vi "相机1-分析PCB孔影像-校准和自动共用.vi"(8 "error in (no error)":errorcluster, 9 "拍照功能":T10, 10 "取像时间":u32, 11 "Image In":T12) -> (0 "error out":errorcluster, 1 "Mark点拍照结果":bool=TRUE, 2 "mark Angle":sgl, 3 "Image":T12(plugin-control), 4 "存档数据和结果 out":T9={"待写入数据"=[], "单个结果"=[], "总结果"=FALSE, "数据有效"=TRUE}, 5 "视觉补偿机械手移动量 mm":T11 {"X" format="%#.3f"})   [LabVIEW 2014]
uses:
  <vilib>/vision/Image Controls.llb/IMAQ Image.ctl
  Controls/XYPos.ctl
  <vilib>/vision/Instrument.llb/QR Code Report.ctl
  <vilib>/vision/Instrument.llb/QR Code Model Type.ctl
  <vilib>/vision/Instrument.llb/QR Code Stream Mode Type.ctl
  <vilib>/vision/Instrument.llb/Data Matrix Polarity.ctl
  <vilib>/vision/Instrument.llb/Demodulation Mode.ctl
  <vilib>/vision/Instrument.llb/Cell Sample Size.ctl
  <vilib>/vision/Instrument.llb/Cell Filter Mode.ctl
  Controls/TestThreshold.ctl
  <vilib>/vision/Measure.llb/Edge Options.ctl
  <vilib>/vision/Measure.llb/Edge Polarity.ctl
  Global.vi
  <vilib>/vision/NI_Vision_Development_Module.lvlib
panel:
  out "QR Barcode Report (2D Barcode Reader 1)":T1={"Found?"=FALSE, "Data"="", "Bounding Box"=[], "Errors Corrected"=0, "Dimensions (Rows/Cols)"=0, "Version"=0, "QR Model"=3, "Stream Mode"=0, "Barcode Polarity"=-2, "Mirrored?"=FALSE, "Append Stream Position"=0, "Size of Append Stream"=0, "First EAN-128 ID"=0, "First Alternate Language ID"=0, "Append Stream ID"=0, "Minimum Edge Strength"=30, "Demodulation Mode"=-2, "Cell Sample Size"=-2, "Cell Filter Mode"=-2} {"Append Stream ID" format="%x"; "Cell Filter Mode" items=["Auto-detect"=-2, "Average"=0, "Median"=1, "Central Average"=2, "High Average"=3, "Low Average"=4, "Very High Average"=5, "Very Low Average"=6, "All Filters"=8]; "Cell Sample Size" items=["Auto-detect"=-2, "1x1"=1, "2x2"=2, "3x3"=3, "4x4"=4, "5x5"=5, "6x6"=6, "7x7"=7]; "Demodulation Mode" items=["Auto-detect"=-2, "Histogram"=0, "Local Contrast"=1, "Combination"=2, "All"=3]; "Barcode Polarity" items=["Auto-detect"=-2, "Black on White"=0, "White on Black"=1]; "Stream Mode" items=["Auto-detect", "Numeric", "AlphaNumeric", "Mixed", "Raw Bytes", "UCC/EAN-128 - In Tokens", "UCC/EAN-128 - In Data", "Extended Character Interpretation", "Kanji"]; "QR Model" items=["Auto Detect", "Micro", "Model 1", "Model 2"]; "Version" max=40 step=1}
  out "Fitted Circle 2":T8 {"Average SNR (dB)" format="%.2f"; "Average Strength" format="%.2f"; "Roundness (Real-World)" format="%.2f"; "Radius (Real-World)" format="%.2f"; "Center (Real-World)"."Y" format="%.2f"; "Center (Real-World)"."X" format="%.2f"; "Radius (Pixels)" format="%.2f"; "Center (Pixels)"."Y" format="%.2f"; "Center (Pixels)"."X" format="%.2f"}
  out "Fitted Circle":T8 {"Average SNR (dB)" format="%.2f"; "Average Strength" format="%.2f"; "Roundness (Real-World)" format="%.2f"; "Radius (Real-World)" format="%.2f"; "Center (Real-World)"."Y" format="%.2f"; "Center (Real-World)"."X" format="%.2f"; "Radius (Pixels)" format="%.2f"; "Center (Pixels)"."Y" format="%.2f"; "Center (Pixels)"."X" format="%.2f"}
  in  "存档数据和结果":T9={"待写入数据"=[], "单个结果"=[], "总结果"=FALSE, "数据有效"=TRUE}
  in  "显示内容 2":string[](array[string])=["补偿量-X", "补偿量-Y", "补偿量-角度"]
  out "图像偏差量Pixles":T11 {"X" format="%#.3f"}
  in  "Img Path":path=path "C:/Users/aicter/Desktop/上相机对位时Gold影像.png"
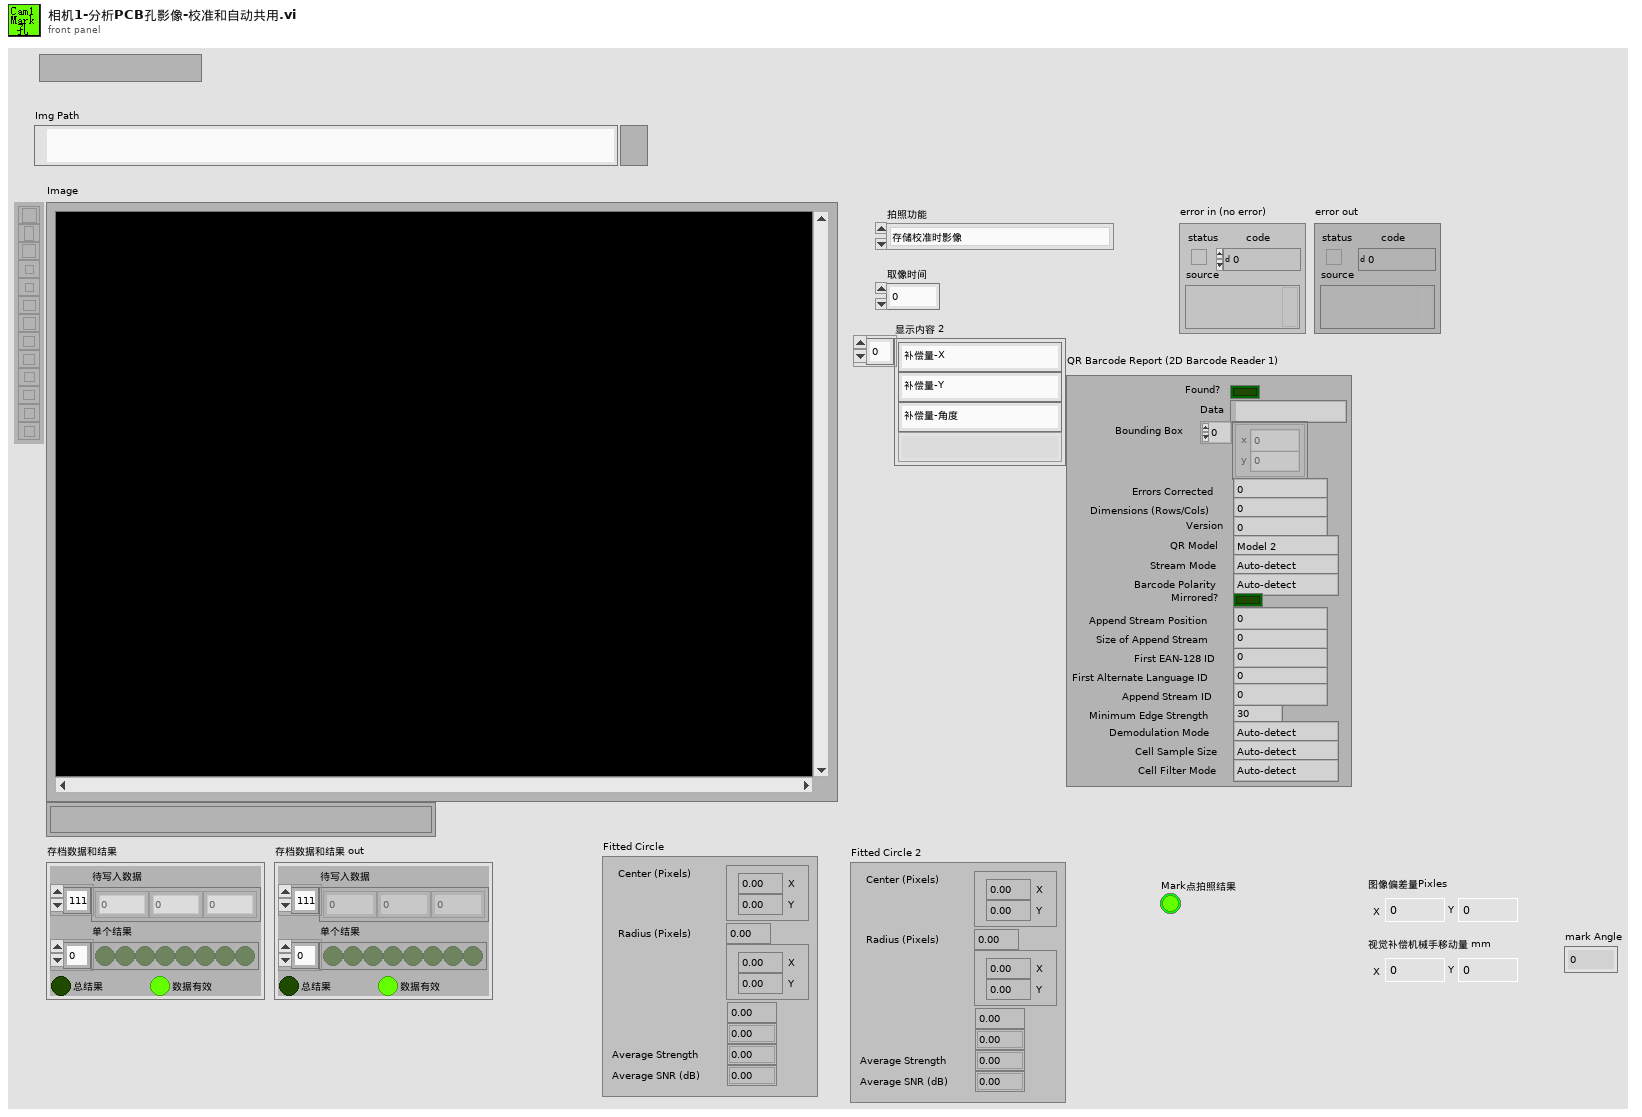
[diagram p1: front panel]
types:
  T1 = typedef "QR Code Report.ctl" = cluster{"Found?":bool, "Data":string, "Bounding Box":cluster{"x":sgl, "y":sgl}[], "Errors Corrected":u32, "Dimensions (Rows/Cols)":u32, "Version":u32, "QR Model":T2, "Stream Mode":T3, "Barcode Polarity":T4, "Mirrored?":bool, "Append Stream Position":u32, "Size of Append Stream":u32, "First EAN-128 ID":i32, "First Alternate Language ID":i32, "Append Stream ID":u32, "Minimum Edge Strength":u32, "Demodulation Mode":T5, "Cell Sample Size":T6, "Cell Filter Mode":T7}
  T2 = typedef "QR Code Model Type.ctl" = i32
  T3 = typedef "QR Code Stream Mode Type.ctl" = i32
  T4 = typedef "Data Matrix Polarity.ctl" = i32
  T5 = typedef "Demodulation Mode.ctl" = i32
  T6 = typedef "Cell Sample Size.ctl" = i32
  T7 = typedef "Cell Filter Mode.ctl" = i32
  T8 = cluster{"Center (Pixels)":cluster{"X":sgl, "Y":sgl}, "Radius (Pixels)":dbl, "Center (Real-World)":cluster{"X":sgl, "Y":sgl}, "Radius (Real-World)":dbl, "Roundness (Real-World)":dbl, "Average Strength":dbl, "Average SNR (dB)":dbl}
  T9 = typedef "存档数据和结果.ctl" = cluster{"待写入数据":dbl[], "单个结果":bool[], "总结果":bool, "数据有效":bool}
  T10 = typedef "控件-拍照PCB孔分类.ctl" = enum16{"存储校准时影像", "拍照孔-Mark1", "拍照孔-Mark2", "拍照二维码", "计算补偿量"}
  T11 = typedef "XYPos.ctl" = cluster{"X":dbl, "Y":dbl}
  T12 = typedef "IMAQ Image.ctl" = refnum<image>
  T13 = typedef "Edge Options.ctl" = cluster{"Edge Polarity":T14, "Kernel Size":u32, "Width":u32, "Minimum Edge Strength":sgl, "Interpolation Type":enum32{"Zero Order", "Bilinear", "Quadratic", "Cubic", "Bilinear Fixed"}, "Data Processing Method":enum32{"Average", "Median"}}
  T14 = typedef "Edge Polarity.ctl" = u32
  T15 = cluster{"Search  Direction":u32, "Edge Options":T13, "Show Search Area":bool, "Show Search Lines":bool, "Show Edges Found":bool, "Show Result":bool, "Search Area Color":u32, "Search Lines Color":u32, "Edge Locations Color":u32, "Result Color":u32, "Overlay Group Name":string}
  T16 = typedef "TestThreshold.ctl" = cluster{"下限":dbl, "上限":dbl}
  T17 = typedef "OtherSpec.ctl" = cluster{"其它勾选类规格":T18, "其它数据类规格":T19, "相机名称":T20, "参数":cluster{"Mark1曝光时间":i32, "Mark2曝光时间":i32, "二维码曝光时间":i32}}
  T18 = typedef "其它勾选类规格.ctl" = cluster{"保存图片":bool, "上传设备状态数据":bool, "保存数据":bool, "开机默认开启监控摄像头":bool, "启用mark拍照 ":bool}
  T19 = typedef "其他数据类规格.ctl" = cluster{"相机1像素-毫米换算系数":dbl, "相机2像素-毫米换算系数":dbl, "D盘剩余空间预警(G)":dbl, "视频最长录制时间(秒)":dbl}
  T20 = typedef "相机名称品牌使用状态.ctl" = cluster{"相机1名称":T21, "相机2名称":T21, "Cam1启用":bool, "Cam2启用":bool, "Basler1":bool, "Basler2":bool}
  T21 = typedef "IMAQdx.ctl" = refnum<k21>
  T22 = typedef "mark规格.ctl" = cluster{"X下限":dbl, "X上限":dbl, "Y下限":dbl, "Y 上限":dbl, "angle下限":dbl, "angle上限":dbl}
  T23 = cluster{"甩线补偿值":cluster{"下边":dbl, "距离上边":dbl, "左边":dbl, "右边":dbl}, "补偿甩线坐标偏移":T11, "mark点模组补偿":T11, "出线补偿值":dbl, "mark规格":T22}
  T24 = cluster{"mark 1 ":cluster{"X":dbl, "Y":dbl}, "mark 2":cluster{"X":dbl, "Y":dbl}}
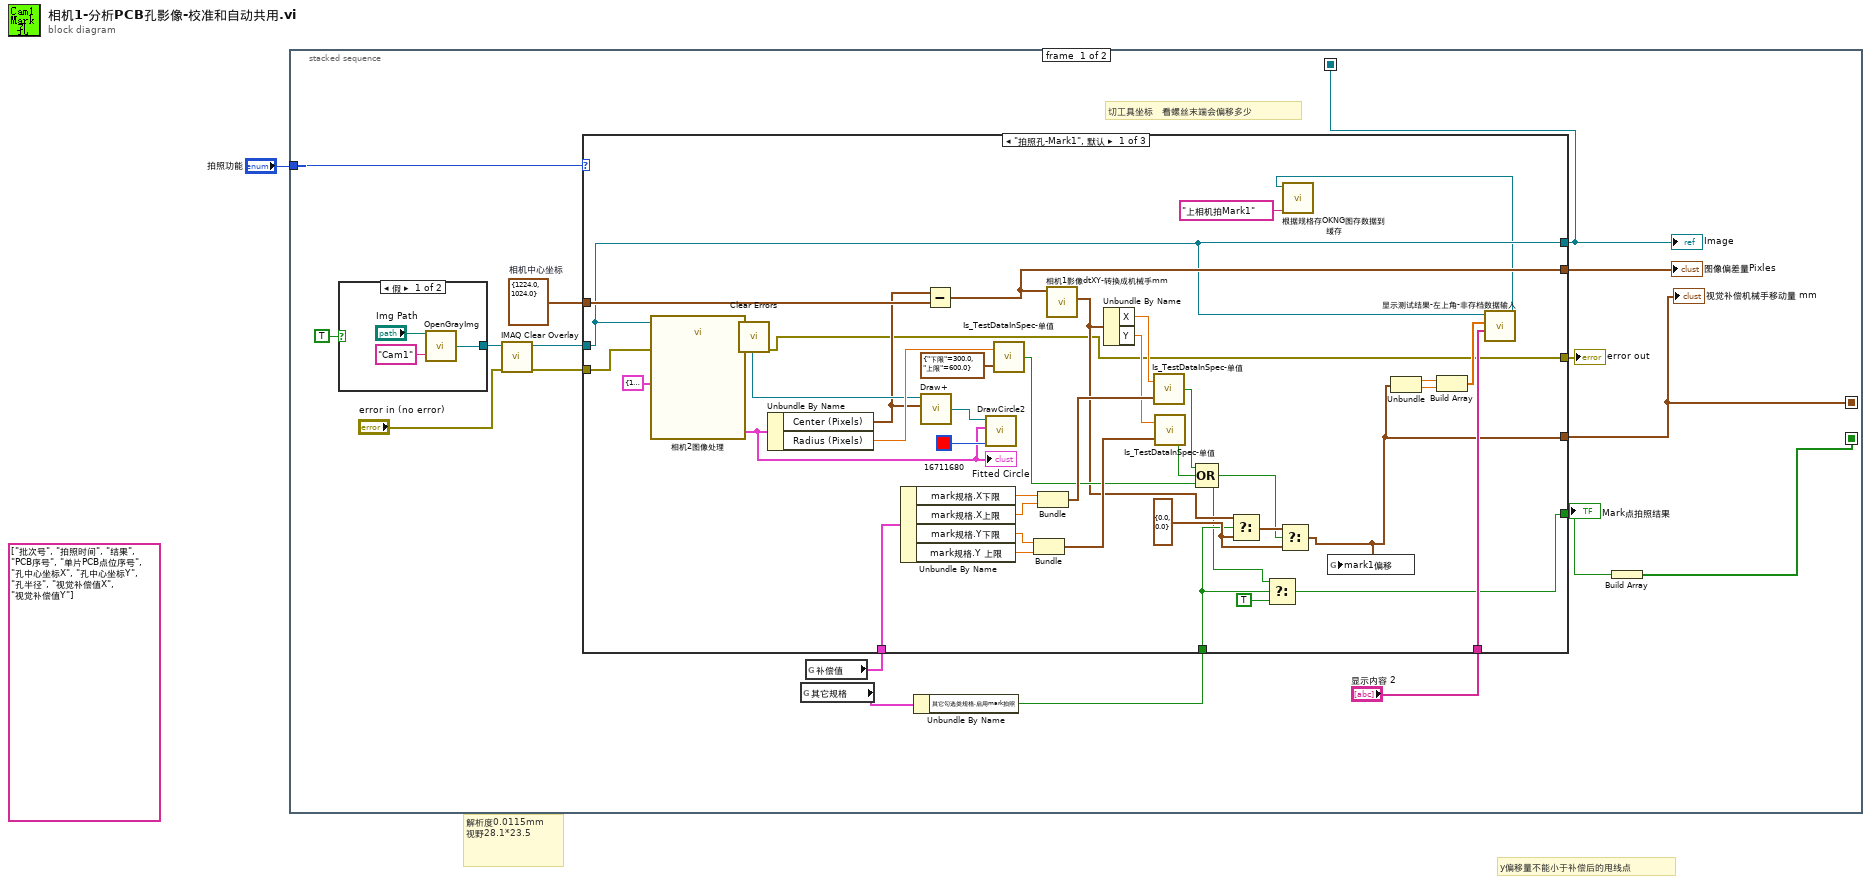
[diagram p0: block diagram]
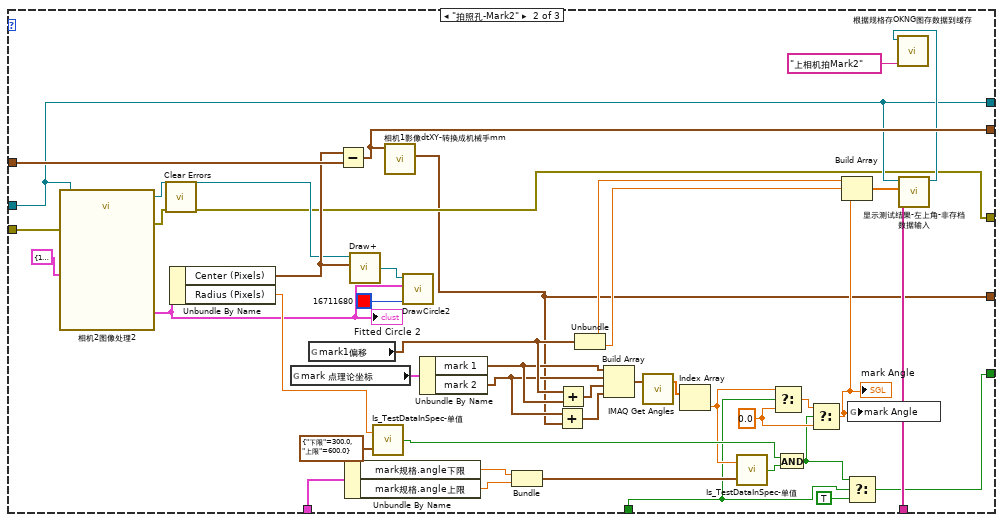
[diagram p2: hidden frame]
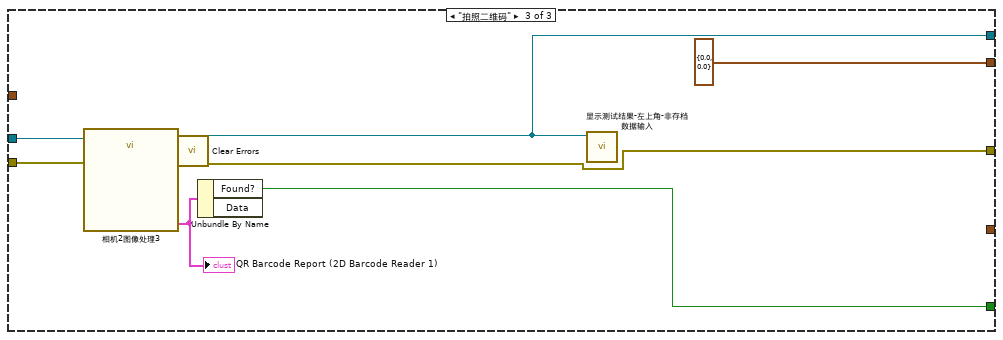
[diagram p3: hidden frame]
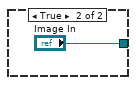
[diagram p4: hidden frame]
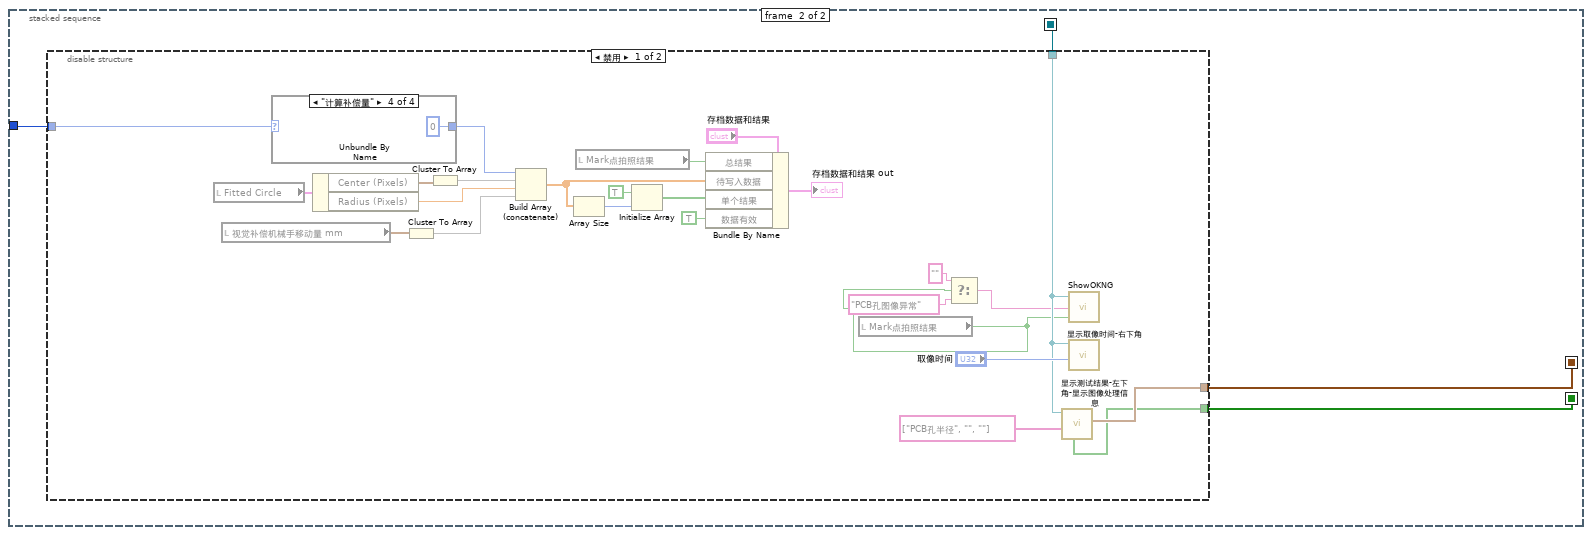
[diagram p5: hidden frame]
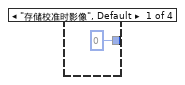
[diagram p6: hidden frame]
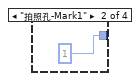
[diagram p7: hidden frame]
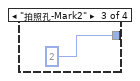
[diagram p8: hidden frame]
diagram:
  (unwired) string[] ["批次号", "拍照时间", "结果", "PCB序号", "单片PCB点位序号", "孔中心坐标X", "孔中心坐标Y", "孔半径", "视觉补偿值X", "视觉补偿值Y"] ("拍PCB孔信息")
  # "y偏移量不能小于补偿后的甩线点"
  # "解析度0.0115mm\n视野28.1*23.5"
  n1 = stacked-sequence {
    seq-local: [w13 _] -> [_ w116]
    seq-local: [w4 _] -> [_ w115]
    seq-local: [w12 _] -> [_ w114]
    tunnel: "拍照功能" -> [w14 w117]
    frame #0 {
      w16 = T11 {"X"=1224.0, "Y"=1024.0}  # 相机中心坐标
      # "切工具坐标   看螺丝末端会偏移多少"
      n2 = case shown="假" TRUE {
        tunnel: [w112 "Image In"] -> w18
        frame False {
          n3 = call "OpenGrayImg.vi"("Image Name"="Cam1", "Img Path"="Img Path") -> ("Image Out"=w112:T12)
        }
        frame True {
        }
      }
      n4 = call "IMAQ Clear Overlay"("error in (no error)"="error in (no error)", "Image"=w18) -> ("error out"=w8:errorcluster, "Image Out"=w7:T12)  [unwired: 8 in]
      n5 = global read "Global.vi" "其它规格"() -> (w11:T17)
      n6 = global read "Global.vi" "补偿值"() -> (w3:T23)
      n7 = Unbundle By Name(w11) -> ("其它勾选类规格.启用mark拍照"=w2:bool)
      n8 = case shown="\"拍照孔-Mark1\", 默认" w14 {
        tunnel: w7 -> [w48 w65 w108]
        tunnel: w16 -> [w58 w100 _]
        tunnel: [w48 w65 w105] -> w13
        tunnel: [w57 w99 T11 {"X"=0.0, "Y"=0.0} ("相机中心坐标")] -> w15
        tunnel: "显示内容 2" -> [w55 w97 _]
        tunnel: w8 -> [w46 w64 w109]
        tunnel: [w20 w60 w102] -> w6
        tunnel: [w23 w68 w103] -> w5
        tunnel: [w19 w59 _] -> w4
        tunnel: w3 -> [w32 w86 _]
        tunnel: w2 -> [w24 w70 _]
        frame "拍照孔-Mark1", Default {
          w29 = T11 {"X"=0.0, "Y"=0.0} ("f")
          n9 = call "相机2图像处理"("Image In"=w48, "Options (Find Circular Edge 1)"=T15 {"Search  Direction"=1, "Edge Options"={"Edge Polarity"=1, "Kernel Size"=9, "Width"=5, "Minimum Edge Strength"=30.0, "Interpolation Type"=enum."Bilinear Fixed", "Data Processing Method"=enum."Average"}, "Show Search Area"=FALSE, "Show Search Lines"=FALSE, "Show Edges Found"=TRUE, "Show Result"=FALSE, "Search Area Color"=65280, "Search Lines Color"=255, "Edge Locations Color"=16776960, "Result Color"=16711680, "Overlay Group Name"=""}, "error in"=w46) -> ("Image Out"=w47:T12, "Fitted Circle (Find Circular Edge 1)"=w52:T8, "error out"=w44:errorcluster)  [unwired: 21 in, 1 out]
          "Fitted Circle" <- w52
          n10 = call <vilib>:"Clear Errors.vi"("error in (no error)"=w44) -> ("error out"=w20:errorcluster)  [unwired: 5 in, 1 out]
          n11 = Unbundle By Name(w52) -> ("Center (Pixels)"=w45:cluster{"X":sgl, "Y":sgl}, "Radius (Pixels)"=w50:dbl)
          n12 = Unbundle By Name(w32) -> ("mark规格.X下限"=w42:dbl, "mark规格.X上限"=w41:dbl, "mark规格.Y下限"=w38:dbl, "mark规格.Y 上限"=w37:dbl)
          n13 = call "Draw+.vi"("input cluster"=w45, "Image In"=w47) -> ("Image Out"=w54:T12)  [unwired: 4 in]
          n14 = Subtract(x=w45, y=w58) -> (x-y=w57:T11)
          n15 = call "DrawCircle2.vi"("Color"=u32 16711680, "Fitted Circle (左圆)"=w52, "Img in"=w54) -> ()  [unwired: 1 in, 1 out]
          n16 = call "Is_TestDataInSpec-单值.vi"("量测规格"=T16 {"下限"=300.0, "上限"=600.0}, "相机量测结果"=w50) -> ("在规格内"=w35:bool)
          n17 = Bundle("Y下限"=w38, "Y 上限"=w37) -> (w36:cluster{"Y下限":dbl, "Y 上限":dbl})  [unwired: 1 in]
          n18 = Bundle("X下限"=w42, "X上限"=w41) -> (w40:cluster{"X下限":dbl, "X上限":dbl})  [unwired: 1 in]
          n19 = call "相机1影像dtXY-转换成机械手mm.vi"("校准：相机1示教时影像坐标"=w57) -> ("机械手移动量 mm"=w31:T11)  [unwired: 9 in, 1 out]
          n20 = Unbundle By Name(w31) -> ("X"=w43:dbl, "Y"=w39:dbl)
          n21 = call "Is_TestDataInSpec-单值.vi"("量测规格"=w40, "相机量测结果"=w43) -> ("在规格内"=w34:bool)
          n22 = call "Is_TestDataInSpec-单值.vi"("量测规格"=w36, "相机量测结果"=w39) -> ("在规格内"=w33:bool)
          n23 = Compound Arithmetic op=OR(w34, w33, w35) -> (w21:bool)
          n24 = Select(t=w31, s=w24, f=w29) -> (s? t:f=w30:T11)
          n25 = Select(t=w21, s=w24, f=TRUE) -> (s? t:f=w23:bool)
          n26 = Select(t=w30, s=w21, f=w29) -> (s? t:f=w19:T11)
          n27 = global write "Global.vi" "mark1偏移"(w19) -> ()
          n28 = Unbundle(w19) -> ("X"=w27:dbl, "Y"=w26:dbl)
          n29 = Build Array(w27, w26) -> (w25:dbl[])
          n30 = call "显示测试结果-左上角-非存档数据输入.vi"("量测项目名称"=w55, "显示数据"=w25, "Img输入"=w48) -> ("Image Out"=w28:T12)  [unwired: 8 in]
          n31 = call "根据规格存OKNG图存数据到缓存.vi"("选择相机字符串"="上相机拍Mark1", "Img输入"=w28) -> ()  [unwired: 10 in]
        }
        frame "拍照孔-Mark2" {
          w72 = sgl 0.0 ("f")
          n32 = call "相机2图像处理2"("Image In"=w65, "Options (Find Circular Edge 1)"=T15 {"Search  Direction"=1, "Edge Options"={"Edge Polarity"=1, "Kernel Size"=9, "Width"=5, "Minimum Edge Strength"=30.0, "Interpolation Type"=enum."Bilinear Fixed", "Data Processing Method"=enum."Average"}, "Show Search Area"=FALSE, "Show Search Lines"=FALSE, "Show Edges Found"=TRUE, "Show Result"=FALSE, "Search Area Color"=65280, "Search Lines Color"=255, "Edge Locations Color"=16776960, "Result Color"=16711680, "Overlay Group Name"=""}, "error in"=w64) -> ("Image Out"=w63:T12, "Fitted Circle (Find Circular Edge 1)"=w61:T8, "error out"=w62:errorcluster)  [unwired: 21 in, 1 out]
          "Fitted Circle 2" <- w61
          n33 = call <vilib>:"Clear Errors.vi"("error in (no error)"=w62) -> ("error out"=w60:errorcluster)  [unwired: 5 in, 1 out]
          n34 = Unbundle By Name(w61) -> ("Center (Pixels)"=w92:cluster{"X":sgl, "Y":sgl}, "Radius (Pixels)"=w93:dbl)
          n35 = global read "Global.vi" "mark 点理论坐标"() -> (w91:T24)
          n36 = global read "Global.vi" "mark1偏移"() -> (w79:T11)
          n37 = Subtract(x=w92, y=w100) -> (x-y=w99:T11)
          n38 = Unbundle By Name(w86) -> ("mark规格.angle下限"=w85:dbl, "mark规格.angle上限"=w84:dbl)
          n39 = call "Draw+.vi"("input cluster"=w92, "Image In"=w63) -> ("Image Out"=w96:T12)  [unwired: 4 in]
          n40 = call "Is_TestDataInSpec-单值.vi"("量测规格"=T16 {"下限"=300.0, "上限"=600.0}, "相机量测结果"=w93) -> ("在规格内"=w82:bool)
          n41 = call "相机1影像dtXY-转换成机械手mm.vi"("校准：相机1示教时影像坐标"=w99) -> ("机械手移动量 mm"=w59:T11)  [unwired: 9 in, 1 out]
          n42 = call "DrawCircle2.vi"("Color"=u32 16711680, "Fitted Circle (左圆)"=w61, "Img in"=w96) -> ()  [unwired: 1 in, 1 out]
          n43 = Unbundle By Name(w91) -> ("mark 1"=w78:cluster{"X":dbl, "Y":dbl}, "mark 2"=w75:cluster{"X":dbl, "Y":dbl})
          n44 = Bundle("angle下限"=w85, "angle上限"=w84) -> (w83:cluster{"angle下限":dbl, "angle上限":dbl})  [unwired: 1 in]
          n45 = Add(x=w75, y=w59) -> (x+y=w76:T11)
          n46 = Add(x=w79, y=w78) -> (x+y=w77:T11)
          n47 = Unbundle(w79) -> ("X"=w89:dbl, "Y"=w88:dbl)
          n48 = Build Array(w78, w75, w77, w76) -> (w90:T11[])
          n49 = call "IMAQ Get Angles"("Points"=w90) -> ("Angles (deg)"=w87:sgl[])  [unwired: 4 in, 2 out]
          n50 = Index Array(array=w87) -> (element=w74:sgl)  [unwired: 1 in]
          n51 = call "Is_TestDataInSpec-单值.vi"("量测规格"=w83, "相机量测结果"=w74) -> ("在规格内"=w81:bool)
          n52 = Select(t=w74, s=w70, f=w72) -> (s? t:f=w73:sgl)
          n53 = And(x=w82, y=w81) -> (x .and. y?=w69:bool)
          n54 = Select(t=w73, s=w69, f=w72) -> (s? t:f=w80:sgl)
          "mark Angle" <- w80
          n55 = Build Array(w89, w88, w80) -> (w101:dbl[])
          n56 = Select(t=w69, s=w70, f=TRUE) -> (s? t:f=w68:bool)
          n57 = global write "Global.vi" "mark Angle"(w80) -> ()
          n58 = call "显示测试结果-左上角-非存档数据输入.vi"("量测项目名称"=w97, "显示数据"=w101, "Img输入"=w65) -> ("Image Out"=w71:T12)  [unwired: 8 in]
          n59 = call "根据规格存OKNG图存数据到缓存.vi"("选择相机字符串"="上相机拍Mark2", "Img输入"=w71) -> ()  [unwired: 10 in]
        }
        frame "拍照二维码" {
          n60 = call "相机2图像处理3"("Image In"=w108, "error in"=w109) -> ("Image Out"=w105:T12, "QR Barcode Report (2D Barcode Reader 1)"=w106:T1, "error out"=w104:errorcluster)  [unwired: 23 in]
          "QR Barcode Report (2D Barcode Reader 1)" <- w106
          n61 = call <vilib>:"Clear Errors.vi"("error in (no error)"=w104) -> ("error out"=w102:errorcluster)  [unwired: 5 in, 1 out]
          n62 = Unbundle By Name(w106) -> ("Found?"=w103:bool)  [unwired: 1 out]
          n63 = call "显示测试结果-左上角-非存档数据输入.vi"("Img输入"=w105) -> ()  [unwired: 10 in, 1 out]
        }
      }
      "Image" <- w13
      "图像偏差量Pixles" <- w15
      "视觉补偿机械手移动量 mm" <- w4
      "Mark点拍照结果" <- w5
      "error out" <- w6
      n64 = Build Array(w5) -> (w12:bool[])
    }
    frame #1 {
      n65 = disable-structure shown="禁用" {
        disable-tunnel: w117 -> [w137 _]
        disable-tunnel: w116 -> [w125 _]
        disable-tunnel: w115 -> [w124 _]
        disable-tunnel: w114 -> [w123 _]
        frame Disabled {
          n66 = local read "Fitted Circle"() -> (w118:T8)
          n67 = local read "视觉补偿机械手移动量 mm"() -> (w142:T11)
          n68 = case shown="\"计算补偿量\"" w137 {
            tunnel: [0 ("X") 1 ("X") 2 ("X") 0 ("X")] -> w136
            frame "存储校准时影像", Default {
            }
            frame "拍照孔-Mark1" {
            }
            frame "拍照孔-Mark2" {
            }
            frame "计算补偿量" {
            }
          }
          n69 = Unbundle By Name(w118) -> ("Center (Pixels)"=w141:cluster{"X":sgl, "Y":sgl}, "Radius (Pixels)"=w139:dbl)
          n70 = Cluster To Array(cluster=w142) -> (array=w138:dbl[])
          n71 = Cluster To Array(cluster=w141) -> (array=w140:sgl[])
          n72 = Build Array (concatenate)(w136, w140, w139, w138) -> (w132:dbl[])
          n73 = Array Size(array=w132) -> (size(s)=w130:i32)
          n74 = local read "Mark点拍照结果"() -> (w128:bool)
          n75 = Initialize Array(TRUE, w130) -> (w131:bool[])
          n76 = Bundle By Name(cluster="存档数据和结果", "总结果"=w128, "待写入数据"=w132, "单个结果"=w131, "数据有效"=TRUE) -> (→"存档数据和结果 out":T9)
          n77 = local read "Mark点拍照结果"() -> (w119:bool)
          n78 = Select(t="" ("显示消息"), s=w119, f="PCB孔图像异常" ("显示消息")) -> (s? t:f=w120:string)
          n79 = call "显示测试结果-左下角-显示图像处理信息.vi"("每个数据结果"=w123, "量测项目名称"=string[] ["PCB孔半径", "", ""] ("显示内容名称"), "显示数据"=w124, "Img输入"=w125) -> ()  [unwired: 8 in]
          n80 = call "ShowOKNG.vi"("结果"=w119, "显示消息"=w120, "引用句柄输入"=w125) -> ()
          n81 = call "显示取像时间-右下角.vi"("取像时间"="取像时间", "引用句柄输入"=w125) -> ()  [unwired: 9 in, 1 out]
        }
        frame Enabled {
        }
      }
    }
  }
